vi "Raw File Header Text.vi"(8 "error in (no error)":errorcluster, 9 "Type":string, 10 "Raw Data Period":dbl=0.0001024, 11 "FPGA Refnum out":T1) -> (0 "error out":errorcluster, 1 "Date String":string, 2 "concatenated string":string)   [LabVIEW 2020]
doc: "Author: Scott Hannahs <sth@magnet.fsu.edu>\nCopyright 2018 Florida State University, All rights reserved."
uses:
  RT Controls/FPGA SCH Digitizer Ref.ctl
  <vilib>/Utility/error.llb/Error Cluster From Error Code.vi
  <vilib>/rvi/errors/niLvFpgaAdjustHostInterfaceError.vi
  RT Host Globals.vi
  <vilib>/rvi/interface/nirviReadWriteControl/nirviReadWriteControl.xnode
  NiFpgaLv.dll
  <vilib>/rvi/interface/Simulation/niFpgaSimulationCallBeginRW.vi
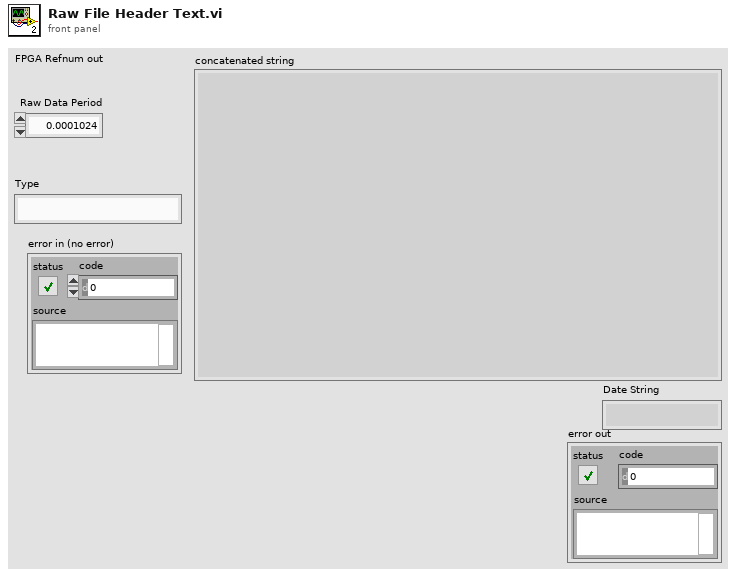
[diagram p1: front panel]
types:
  T1 = typedef "FPGA SCH Digitizer Ref.ctl" = refnum<k20>
  T2 = cluster{"#Coils":u32, "Coil Inductances":fxp<+/-,38,12>[], "Max Coil Currents":fxp<+/-,38,12>[], "Max Coil Volt Dev":fxp<+/-,38,12>[], "Coil A Coefficients":fxp<+/-,38,12>[], "Coil B Coefficients":fxp<+/-,38,12>[], "Coil C Coefficients":fxp<+/-,38,12>[], "Coil D Coefficients":fxp<+/-,38,12>[], "Max Coil Temp":fxp<+/-,38,12>[], " Pressure Range":fxp<+/-,38,12>[], "Temp Coef":fxp<+/-,38,12>[], "Offsets":fxp<+/-,38,12>[], "Scale Factors":fxp<+/-,38,12>[]}
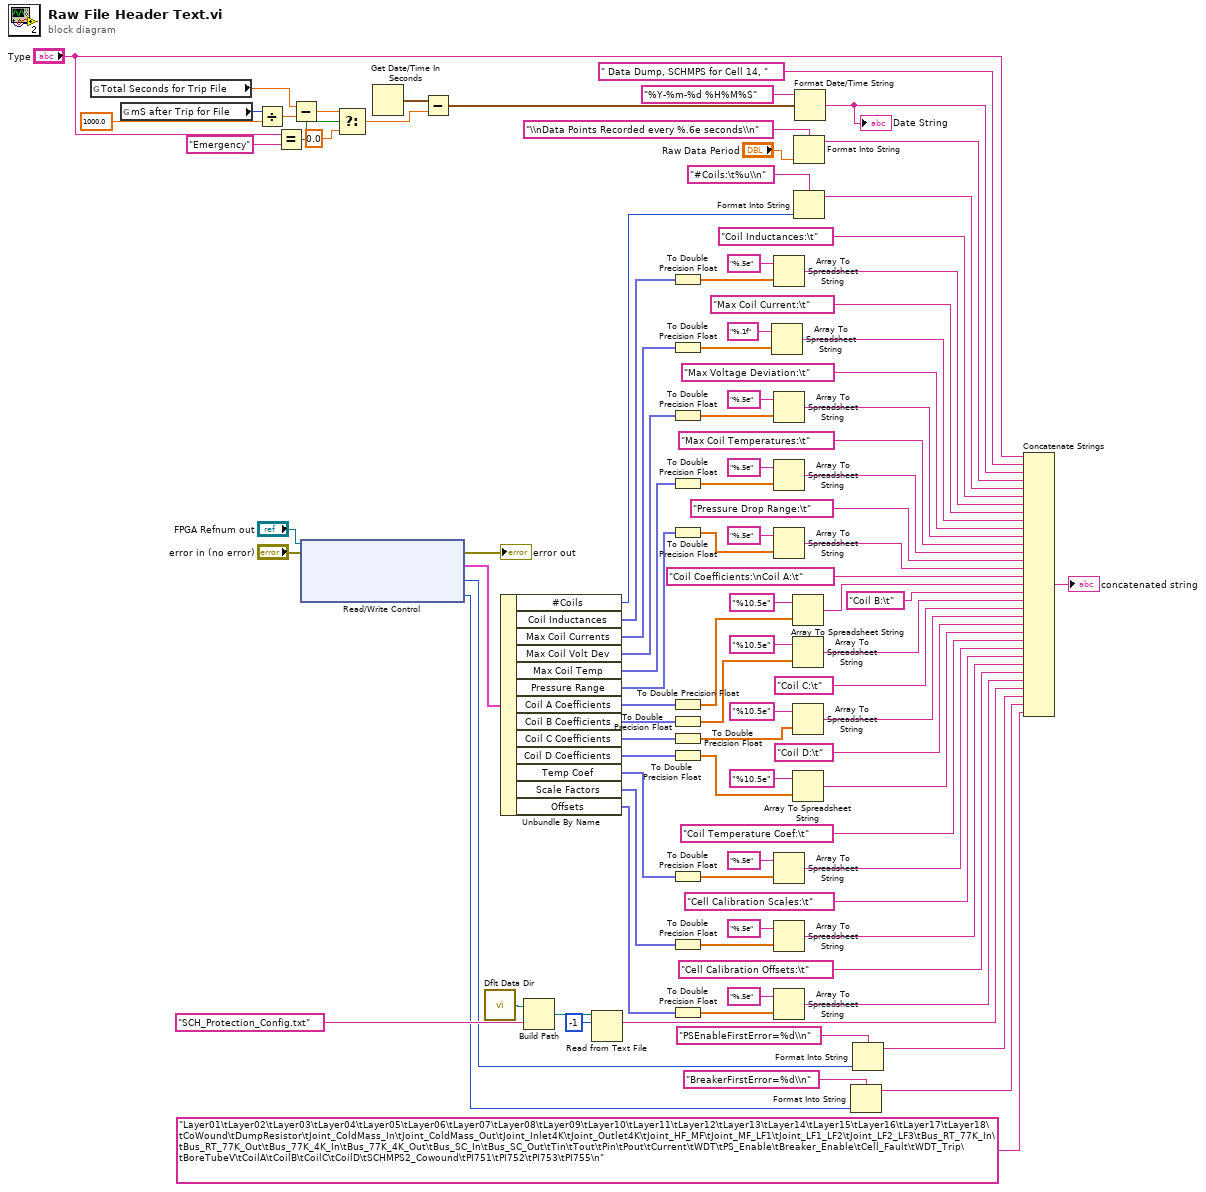
[diagram p0: block diagram]
diagram:
  n1 = global read "RT Host Globals.vi" "Total Seconds for Trip File"() -> (w9:dbl)
  n2 = global read "RT Host Globals.vi" "mS after Trip for File"() -> (w11:u32)
  n3 = Divide(x=w11, y=1000.0) -> (x/y=w8:dbl)
  n4 = Equal?(x="Type", y="Emergency") -> (x = y?=w7:bool)
  n5 = Subtract(x=w9, y=w8) -> (x-y=w3:dbl)
  n6 = xnode "Read/Write Control"("FPGA VI Reference In"="FPGA Refnum out", "error in"="error in (no error)") -> ("error out"=→"error out":errorcluster, "Magnet Configuration Data"=w96:T2, "PS Enable First Error"=w17:u32, "Breaker First Error"=w15:u64)  [unwired: 1 out]
  n7 = Select(t=w3, s=w7, f=0.0) -> (s? t:f=w6:dbl)
  n8 = Get Date/Time In Seconds() -> (seconds since 1Jan1904=w12:timestamp)
  n9 = Subtract(x=w12, y=w6) -> (x-y=w2:timestamp)
  n10 = call <vilib>:"Dflt Data Dir.vi"() -> ("App:Default Data Directory"=w23:path)
  n11 = Unbundle By Name(w96) -> ("#Coils"=w90:u32, "Coil Inductances"=w86:fxp<+/-,38,12>[], "Max Coil Currents"=w82:fxp<+/-,38,12>[], "Max Coil Volt Dev"=w56:fxp<+/-,38,12>[], "Max Coil Temp"=w81:fxp<+/-,38,12>[], "Pressure Range"=w80:fxp<+/-,38,12>[], "Coil A Coefficients"=w79:fxp<+/-,38,12>[], "Coil B Coefficients"=w78:fxp<+/-,38,12>[], "Coil C Coefficients"=w77:fxp<+/-,38,12>[], "Coil D Coefficients"=w76:fxp<+/-,38,12>[], "Temp Coef"=w75:fxp<+/-,38,12>[], "Scale Factors"=w74:fxp<+/-,38,12>[], "Offsets"=w73:fxp<+/-,38,12>[])
  n12 = Build Path(base path=w23, name or relative path="SCH_Protection_Config.txt") -> (appended path=w21:path)
  n13 = Read from Text File(file (use dialog)=w21, count=-1) -> (text=w19:string)  [unwired: 2 in, 3 out]
  n14 = To Double Precision Float(number=w86) -> (double precision float=w85:dbl[])
  n15 = To Double Precision Float(number=w82) -> (double precision float=w72:dbl[])
  n16 = To Double Precision Float(number=w56) -> (double precision float=w63:dbl[])
  n17 = To Double Precision Float(number=w81) -> (double precision float=w62:dbl[])
  n18 = To Double Precision Float(number=w80) -> (double precision float=w61:dbl[])
  n19 = To Double Precision Float(number=w79) -> (double precision float=w51:dbl[])
  n20 = To Double Precision Float(number=w78) -> (double precision float=w50:dbl[])
  n21 = To Double Precision Float(number=w77) -> (double precision float=w49:dbl[])
  n22 = To Double Precision Float(number=w76) -> (double precision float=w48:dbl[])
  n23 = To Double Precision Float(number=w75) -> (double precision float=w32:dbl[])
  n24 = To Double Precision Float(number=w74) -> (double precision float=w35:dbl[])
  n25 = To Double Precision Float(number=w73) -> (double precision float=w36:dbl[])
  n26 = Array To Spreadsheet String(array=w72, 3:"%.1f" ("format string")) -> (spreadsheet string=w69:string)  [unwired: 1 in]
  n27 = Array To Spreadsheet String(array=w85, 3:"%.5e" ("format string")) -> (spreadsheet string=w71:string)  [unwired: 1 in]
  n28 = Array To Spreadsheet String(array=w63, 3:"%.5e" ("format string")) -> (spreadsheet string=w64:string)  [unwired: 1 in]
  n29 = Array To Spreadsheet String(array=w62, 3:"%.5e" ("format string")) -> (spreadsheet string=w59:string)  [unwired: 1 in]
  n30 = Array To Spreadsheet String(array=w61, 3:"%.5e" ("format string")) -> (spreadsheet string=w57:string)  [unwired: 1 in]
  n31 = Array To Spreadsheet String(array=w32, 3:"%.5e" ("format string")) -> (spreadsheet string=w33:string)  [unwired: 1 in]
  n32 = Array To Spreadsheet String(array=w35, 3:"%.5e" ("format string")) -> (spreadsheet string=w30:string)  [unwired: 1 in]
  n33 = Array To Spreadsheet String(array=w36, 3:"%.5e" ("format string")) -> (spreadsheet string=w28:string)  [unwired: 1 in]
  n34 = Array To Spreadsheet String(array=w51, 3:"%10.5e" ("format string")) -> (spreadsheet string=w46:string)  [unwired: 1 in]
  n35 = Array To Spreadsheet String(array=w50, 3:"%10.5e" ("format string")) -> (spreadsheet string=w44:string)  [unwired: 1 in]
  n36 = Array To Spreadsheet String(array=w49, 3:"%10.5e" ("format string")) -> (spreadsheet string=w42:string)  [unwired: 1 in]
  n37 = Array To Spreadsheet String(array=w48, 3:"%10.5e" ("format string")) -> (spreadsheet string=w40:string)  [unwired: 1 in]
  n38 = Format Into String(format string="\\nData Points Recorded every %.6e seconds\\n", "Raw Data Period") -> (resulting string=w93:string)  [unwired: 2 in, 1 out]
  n39 = Format Into String(format string="#Coils:\t%u\\n", w90) -> (resulting string=w88:string)  [unwired: 2 in, 1 out]
  n40 = Format Date/Time String(time format string (%c)="%Y-%m-%d %H%M%S", seconds (now)=w2) -> (date/time string=w24:string)  [unwired: 1 in]
  "Date String" <- w24
  n41 = Format Into String(format string="BreakerFirstError=%d\\n", w15) -> (resulting string=w14:string)  [unwired: 2 in, 1 out]
  n42 = Format Into String(format string="PSEnableFirstError=%d\\n", w17) -> (resulting string=w13:string)  [unwired: 2 in, 1 out]
  n43 = Concatenate Strings("Type", " Data Dump, SCHMPS for Cell 14, ", w24, w93, w88, "Coil Inductances:\t" ("format string"), w71, "Max Coil Current:\t" ("format string"), w69, "Max Voltage Deviation:\t" ("format string"), w64, "Max Coil Temperatures:\t" ("format string"), w59, "Pressure Drop Range:\t" ("format string"), w57, "Coil Coefficients:\nCoil A:\t" ("format string"), w46, "Coil B:\t" ("format string"), w44, "Coil C:\t" ("format string"), w42, "Coil D:\t" ("format string"), w40, "Coil Temperature Coef:\t" ("format string"), w33, "Cell Calibration Scales:\t" ("format string"), w30, "Cell Calibration Offsets:\t" ("format string"), w28, w19, w13, w14, "Layer01\tLayer02\tLayer03\tLayer04\tLayer05\tLayer06\tLayer07\tLayer08\tLayer09\tLayer10\tLayer11\tLayer12\tLayer13\tLayer14\tLayer15\tLayer16\tLayer17\tLayer18\tCoWound\tDumpResistor\tJoint_ColdMass_In\tJoint_ColdMass_Out\tJoint_Inlet4K\tJoint_Outlet4K\tJoint_HF_MF\tJoint_MF_LF1\tJoint_LF1_LF2\tJoint_LF2_LF3\tBus_RT_77K_In\tBus_RT_77K_Out\tBus_77K_4K_In\tBus_77K_4K_Out\tBus_SC_In\tBus_SC_Out\tTin\tTout\tPin\tPout\tCurrent\tWDT\tPS_Enable\tBreaker_Enable\tCell_Fault\tWDT_Trip\tBoreTubeV\tCoilA\tCoilB\tCoilC\tCoilD\tSCHMPS2_Cowound\tPI751\tPI752\tPI753\tPI755\n") -> (→"concatenated string":string)
